vi "_QMH_Close.vi"(8 "error in (no error)":errorcluster, 11 "QMH in":refnum<class "QMH.lvclass">) -> (0 "error out":errorcluster)   [LabVIEW 2018, in "QMH.lvclass"]
uses:
  QMH.lvclass
  QMH.lvclass/QMH.ctl
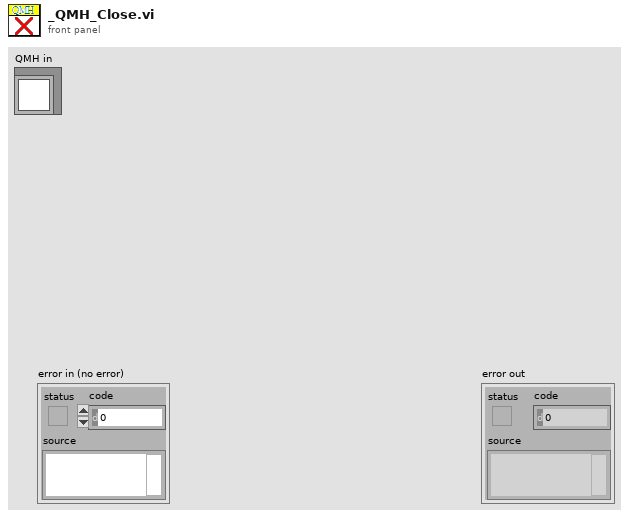
[diagram p1: front panel]
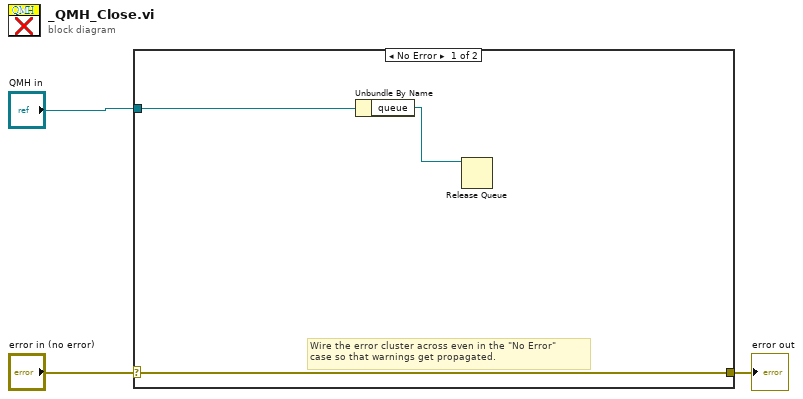
[diagram p0: block diagram]
diagram:
  n1 = case shown="No Error" "error in (no error)" {
    selector: "error in (no error)" -> [w6 w7]
    tunnel: [w6 w7] -> w2
    tunnel: "QMH in" -> [w5 _]
    frame No Error {
      # "Wire the error cluster across even in the \"No Error\"\ncase so that warnings get propagated."
      n2 = Unbundle By Name(w5) -> ("queue"=w4:refnum<queue>)
      n3 = Release Queue(queue=w4) -> ()  [unwired: 2 in, 3 out]
    }
    frame Error {
    }
  }
  "error out" <- w2
